vi "Write Stiffnesses Data.vi"(10 "Stiffnesses Data":T1 {"Forces in Stiffness Summary" min=-888.0 max=888.0; "Stiffnesses in Summary" min=-199630324.20594117 max=199630324.20594117 format="%.2f"; "Displacements in Summary" min=-0.19963032420594115 max=0.19963032420594115 format="%.2f"}, 11 "TestDataLog in":refnum<class "TestDataLog.lvclass">) -> (3 "TestDataLog out":refnum<class "TestDataLog.lvclass">)   [LabVIEW 2015, in "TestDataLog.lvclass"]
uses:
  TestDataLog.lvclass
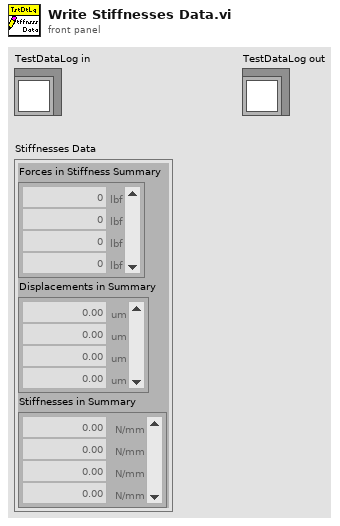
[diagram p1: front panel]
types:
  T1 = cluster{"Forces in Stiffness Summary":dbl[unit][], "Displacements in Summary":dbl[unit][], "Stiffnesses in Summary":dbl[unit][]}
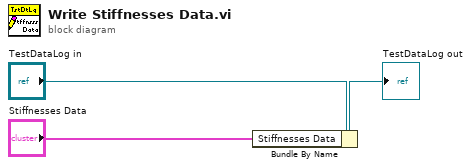
[diagram p0: block diagram]
diagram:
  n1 = Bundle By Name(cluster="TestDataLog in", "Stiffnesses Data"="Stiffnesses Data") -> (→"TestDataLog out":refnum<class "TestDataLog.lvclass">)
